vi "LCOD_UI Control.vi"(6 "Numeric In":i32, 7 "String In":string, 8 "Command":T1) -> (1 "Numeric Out":i32, 2 "String Out":string, 3 "GUI Command Out":T2)   [LabVIEW 2009]
doc: "[Ver 1.00]\nDESCRIPTION\n\nLabVIEW 6.1 version of the LCOD user interface control component. This wraps all required states for the user interface and loads them on the Queue.\n\nINPUTS\nCommand : The actions for this component\nString In : any additional text data that needs passing onto the queue.\nNumeric in : any additional numeric data that needs passing onto the queue.\n\nOUTPUTS\nGUI Command Out : The returned UI state.\nString Out : The returned additional text data\nNumeric Out : The returned additional numeric data\n\nCOMMANDS\nUnder Range : Throws an Error\nGet FP Setting : Returns the UI data from the top of the Queue\n\nUI STATES IN HERE\n\nOver Range : Throws an Error\n\nPRE-CONDITIONS\nCommand-Connection Required\nAll other connections recommended\nUnder Range and Over Range commands generate errors\n\nERROR HANDLING\nThrow error on an Under Range or Over Range command selection.\n\n------------------------------------------------------------------------\n[Ver 1.00]\nSWatts SSDC 03/04/03"
uses:
  LCOD_Stack Queue GUI Command.ctl
  LCOD_FP Command.ctl
  LCOD_Queue Command.ctl
panel:
  # "Output"
  # "Input"
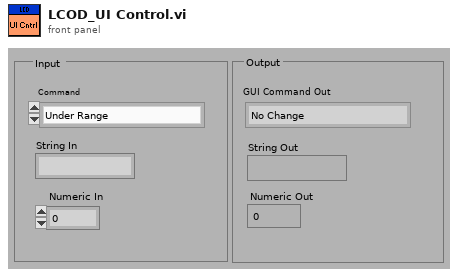
[diagram p1: front panel]
types:
  T1 = typedef "LCOD_FP Command.ctl" = enum16{"Under Range", "Get FP Setting", "HadError", "ResetPressed", "DisplayMsg", "StartPressed", "SetGood", "SetNoGood", "SetIntesting", "Over Range"}
  T2 = typedef "LCOD_Stack Queue GUI Command.ctl" = enum16{"No Change", "HadError", "ResetPressed", "DisplayMsg", "StartPressed", "SetGood", "SetNoGood", "SetIntesting"}
  T3 = typedef "LCOD_Queue Command.ctl" = enum16{"Under Range", "Initialise Stack", "Add To Top", "Add To Bottom", "Pop From Bottom", "More Items?", "Read Bottom", "Over Range"}
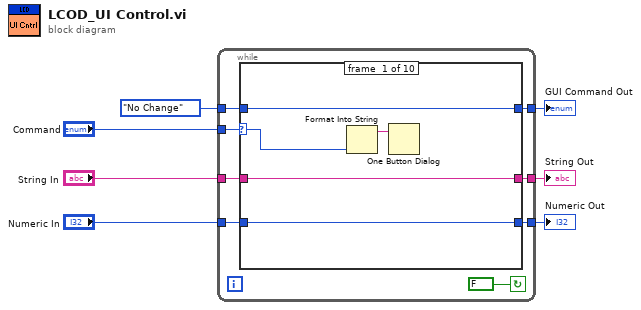
[diagram p0: block diagram]
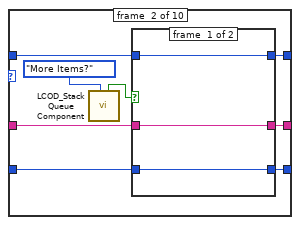
[diagram p2: hidden frame]
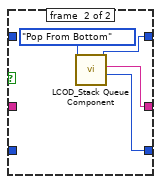
[diagram p3: hidden frame]
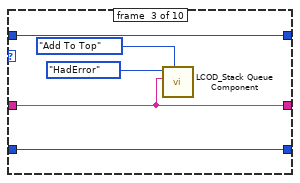
[diagram p4: hidden frame]
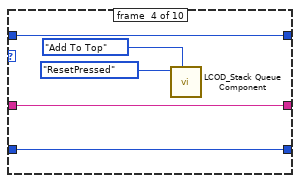
[diagram p5: hidden frame]
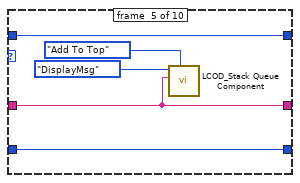
[diagram p6: hidden frame]
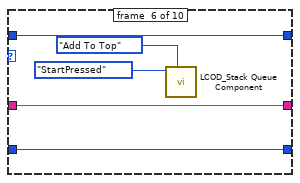
[diagram p7: hidden frame]
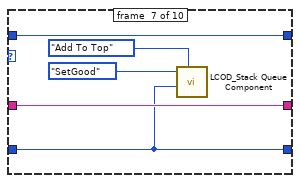
[diagram p8: hidden frame]
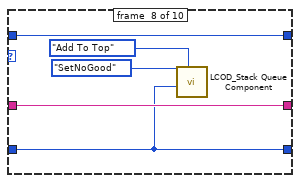
[diagram p9: hidden frame]
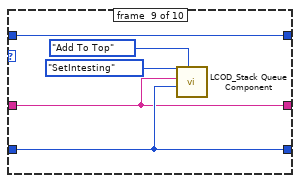
[diagram p10: hidden frame]
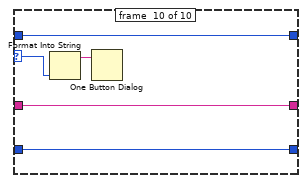
[diagram p11: hidden frame]
diagram:
  n1 = while {
    tunnel: "Command" -> [w8]
    tunnel: LCOD_Stack_Queue_GUI_Command."No Change" ("Command") -> [w15]
    tunnel: [w14] -> w7
    tunnel: [w13] -> w6
    tunnel: [w12] -> w5
    tunnel: "String In" -> [w11]
    tunnel: "Numeric In" -> [w10]
    stop <- FALSE continue-if-true
    n2 = case shown="\"SetIntesting\"" w8 {
      selector: w8 -> [w20 _ _ _ _ _ _ _ _ w74]
      tunnel: w15 -> [w18 w28 w40 w45 w50 w55 w60 w65 w70 w73]
      tunnel: [w18 w27 w40 w45 w50 w55 w60 w65 w70 w73] -> w14
      tunnel: [w17 w26 w36 w44 w46 w54 w59 w64 w66 w72] -> w13
      tunnel: [w16 w25 w39 w43 w49 w53 w58 w63 w69 w71] -> w12
      tunnel: w11 -> [w17 w23 w36 w44 w46 w54 w59 w64 w66 w72]
      tunnel: w10 -> [w16 w24 w39 w43 w49 w53 w58 w63 w69 w71]
      frame #0 {
        n3 = Format Into String(w20) -> (resulting string=w19:string)  [unwired: 3 in, 1 out]
        n4 = One Button Dialog(message=w19) -> ()  [unwired: 2 out]
      }
      frame #1 {
        n5 = call "LCOD_Stack Queue Component.vi"("Command"=LCOD_Queue_Command."More Items?") -> ("More Items?"=w22:bool)  [unwired: 4 in, 4 out]
        n6 = case shown="True" w22 {
          tunnel: w28 -> [w29 _]
          tunnel: [w29 w34] -> w27
          tunnel: [w31 w33] -> w26
          tunnel: [w30 w32] -> w25
          tunnel: w24 -> [w30 _]
          tunnel: w23 -> [w31 _]
          frame #0 {
          }
          frame #1 {
            n7 = call "LCOD_Stack Queue Component.vi"("Command"=LCOD_Queue_Command."Pop From Bottom") -> ("Numeric Out"=w32:i32, "String Out"=w33:string, "GUI Command Out"=w34:T2)  [unwired: 4 in, 2 out]
          }
        }
      }
      frame #2 {
        n8 = call "LCOD_Stack Queue Component.vi"("Command"=LCOD_Queue_Command."Add To Top", "String In"=w36, "GUI Command"=LCOD_Stack_Queue_GUI_Command."HadError" ("Command")) -> ()  [unwired: 2 in, 5 out]
      }
      frame #3 {
        n9 = call "LCOD_Stack Queue Component.vi"("Command"=LCOD_Queue_Command."Add To Top", "GUI Command"=LCOD_Stack_Queue_GUI_Command."ResetPressed" ("Command")) -> ()  [unwired: 3 in, 5 out]
      }
      frame #4 {
        n10 = call "LCOD_Stack Queue Component.vi"("Command"=LCOD_Queue_Command."Add To Top", "String In"=w46, "GUI Command"=LCOD_Stack_Queue_GUI_Command."DisplayMsg" ("Command")) -> ()  [unwired: 2 in, 5 out]
      }
      frame #5 {
        n11 = call "LCOD_Stack Queue Component.vi"("Command"=LCOD_Queue_Command."Add To Top", "GUI Command"=LCOD_Stack_Queue_GUI_Command."StartPressed" ("Command")) -> ()  [unwired: 3 in, 5 out]
      }
      frame #6 {
        n12 = call "LCOD_Stack Queue Component.vi"("Command"=LCOD_Queue_Command."Add To Top", "Numeric In"=w58, "GUI Command"=LCOD_Stack_Queue_GUI_Command."SetGood" ("Command")) -> ()  [unwired: 2 in, 5 out]
      }
      frame #7 {
        n13 = call "LCOD_Stack Queue Component.vi"("Command"=LCOD_Queue_Command."Add To Top", "Numeric In"=w63, "GUI Command"=LCOD_Stack_Queue_GUI_Command."SetNoGood" ("Command")) -> ()  [unwired: 2 in, 5 out]
      }
      frame #8 {
        n14 = call "LCOD_Stack Queue Component.vi"("Command"=LCOD_Queue_Command."Add To Top", "Numeric In"=w69, "String In"=w66, "GUI Command"=LCOD_Stack_Queue_GUI_Command."SetIntesting" ("Command")) -> ()  [unwired: 1 in, 5 out]
      }
      frame #9 {
        n15 = Format Into String(w74) -> (resulting string=w75:string)  [unwired: 3 in, 1 out]
        n16 = One Button Dialog(message=w75) -> ()  [unwired: 2 out]
      }
    }
  }
  "GUI Command Out" <- w7
  "String Out" <- w6
  "Numeric Out" <- w5
